vi "CallCheckIdle.vi"(6 "Time out?":u8, 8 "error in (no error)":errorcluster, 11 "FPGA VI引用输入":refnum<k20>) -> (0 "error out":errorcluster, 3 "FPGA VI引用输出":refnum<k20>)   [LabVIEW 2015]
uses:
  <vilib>/Utility/error.llb/Error Cluster From Error Code.vi
  <vilib>/rvi/errors/niLvFpgaAdjustHostInterfaceError.vi
  <vilib>/rvi/interface/nirviReadWriteControl/nirviReadWriteControl.xnode
  NiFpgaLv.dll
  <vilib>/rvi/interface/Simulation/niFpgaSimulationCallBeginRW.vi
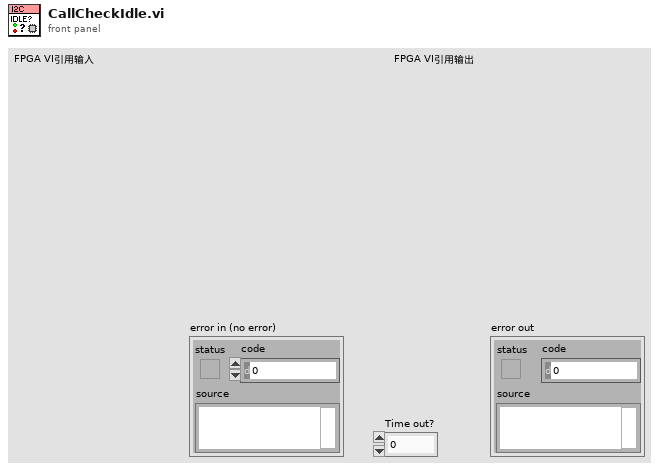
[diagram p1: front panel]
types:
  T1 = enum8{"IDLE", "SetIDLE", "Config", "Arm", "Read", "Write", "AutoRead"}
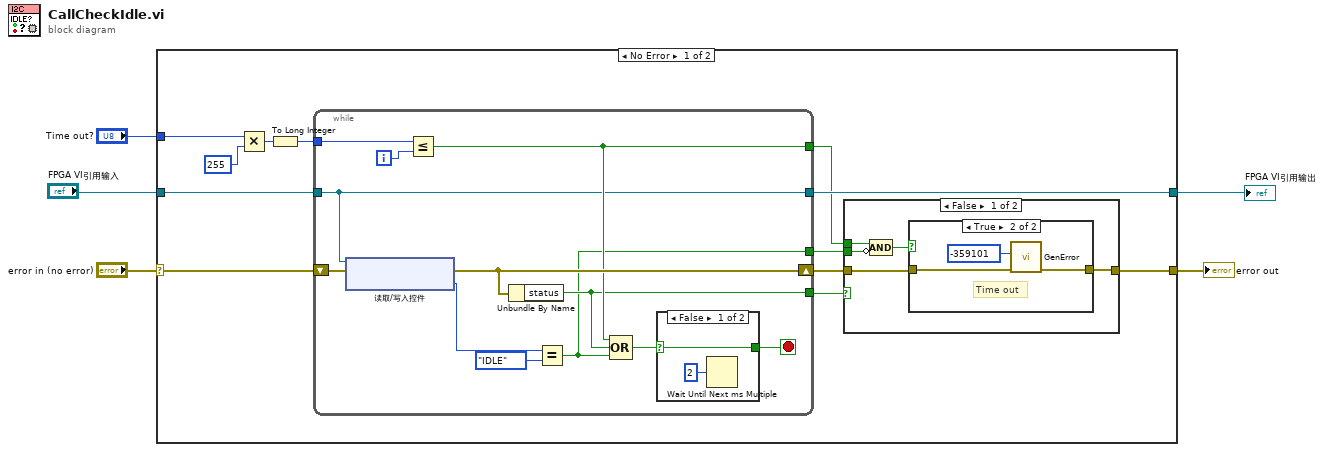
[diagram p0: block diagram]
diagram:
  n1 = case shown="No Error" "error in (no error)" {
    selector: "error in (no error)" -> [w16 w44]
    tunnel: [w17 w44] -> w5
    tunnel: "Time out?" -> [w13 _]
    tunnel: "FPGA VI引用输入" -> [w15 w43]
    tunnel: [w14 w43] -> w1
    frame No Error {
      n2 = Multiply(x=w13, y=u8 255) -> (x*y=w6:u8)
      n3 = To Long Integer(number=w6) -> (32bit integer=w11:i32)
      n4 = while {
        shift-right: [w36] -> w10
        shift-left: w16 -> [w39]
        tunnel: [w30] -> w14
        tunnel: w15 -> [w30]
        tunnel: w11 -> [w37]
        tunnel: [w35] -> w7
        tunnel: [w31] -> w8
        tunnel: [w32] -> w9
        i -> [w38]
        stop <- w33 stop-if-true
        n5 = xnode "读取/写入控件"("FPGA VI Reference In"=w30, "error in"=w39) -> ("error out"=w36:errorcluster, "ProtocolControl"=w29:T1)  [unwired: 1 out]
        n6 = Less Or Equal?(x=w37, y=w38) -> (x <= y?=w35:bool)
        n7 = Unbundle By Name(w36) -> ("status"=w32:bool)
        n8 = Equal?(x=w29, y=T1."IDLE") -> (x = y?=w31:bool)
        n9 = Compound Arithmetic op=OR(w35, w32, w31) -> (w34:bool)
        n10 = case shown="False" w34 {
          selector: w34 -> [w41 w42]
          tunnel: [w41 w42] -> w33
          frame False {
            n11 = Wait Until Next ms Multiple(millisecond multiple=u32 2) -> ()  [unwired: 1 out]
          }
          frame True {
          }
        }
      }
      n12 = case shown="False" w9 {
        tunnel: w10 -> [w22 w27]
        tunnel: [w21 w27] -> w17
        tunnel: w8 -> [w20 _]
        tunnel: w7 -> [w18 _]
        frame False {
          n13 = Compound Arithmetic op=AND(w18, invert w20) -> (w19:bool)
          n14 = case shown="True" w19 {
            tunnel: w22 -> [w23 w26]
            tunnel: [w23 w25] -> w21
            frame False {
            }
            frame True {
              # "Time out"
              n15 = call "GenError.vi"("error in (no error)"=w26, "Code"=-359101) -> ("error out"=w25:errorcluster)  [unwired: 9 in]
            }
          }
        }
        frame True {
        }
      }
    }
    frame Error {
    }
  }
  "error out" <- w5
  "FPGA VI引用输出" <- w1
